vi "FindNextMultipleOfN.vi"(1 "Input":i32, 2 "n":i32) -> (0 "Integer":i32)   [LabVIEW 2012, in "NFC Driver.lvlib"]
doc: "This VI converts a raw HEX string into it's ASCII representation"
uses:
  NFC Driver.lvlib
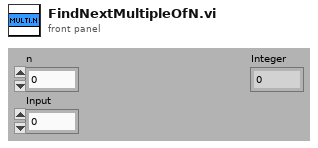
[diagram p1: front panel]
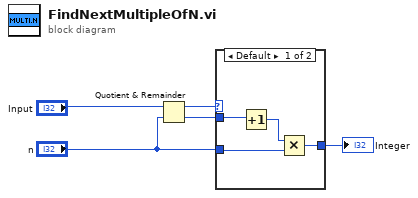
[diagram p0: block diagram]
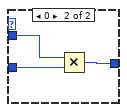
[diagram p2: hidden frame]
diagram:
  n1 = Quotient & Remainder(x="Input", y="n") -> (x-y*floor(x/y)=w4:i32, floor(x/y)=w3:i32)
  n2 = case shown="Default" w4 {
    tunnel: w3 -> [w9 w12]
    tunnel: "n" -> [w7 w11]
    tunnel: [w6 w10] -> w1
    frame Default {
      n3 = Increment(x=w9) -> (x+1=w8:i32)
      n4 = Multiply(x=w8, y=w7) -> (x*y=w6:i32)
    }
    frame 0 {
      n5 = Multiply(x=w12, y=w11) -> (x*y=w10:i32)
    }
  }
  "Integer" <- w1
